vi "Update MLBox.vi"(8 "error in (no error)":errorcluster, 11 "Table View in":refnum<class "Table View.lvclass">) -> (0 "error out":errorcluster, 3 "Table View out":refnum<class "Table View.lvclass">)   [LabVIEW 2020, in "[V]Table View.lvlib" / "Table View.lvclass"]
uses:
  Table View.lvclass
  <vilib>/HUASUI/MulListBox/Type Definitions/Autosize Mode.ctl
  Table View.lvclass/Table View.ctl
  <vilib>/HUASUI/MulListBox/MListBox.lvclass/MListBox.ctl
  <vilib>/HUASUI/MulListBox/MListBox.lvclass
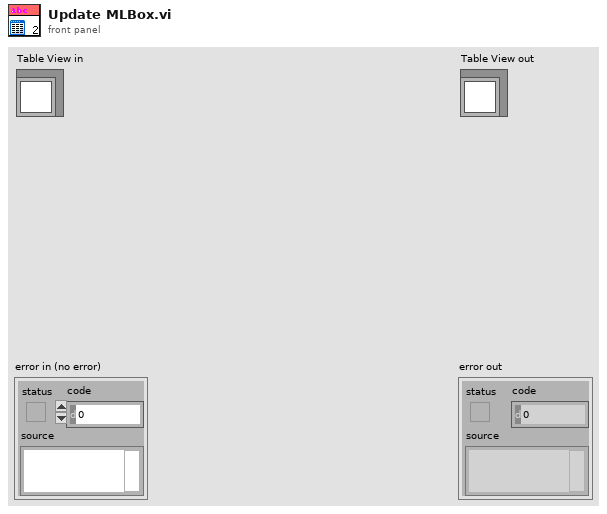
[diagram p1: front panel]
types:
  T1 = typedef "Autosize Mode.ctl" = enum16{"Header", "All Cells"}
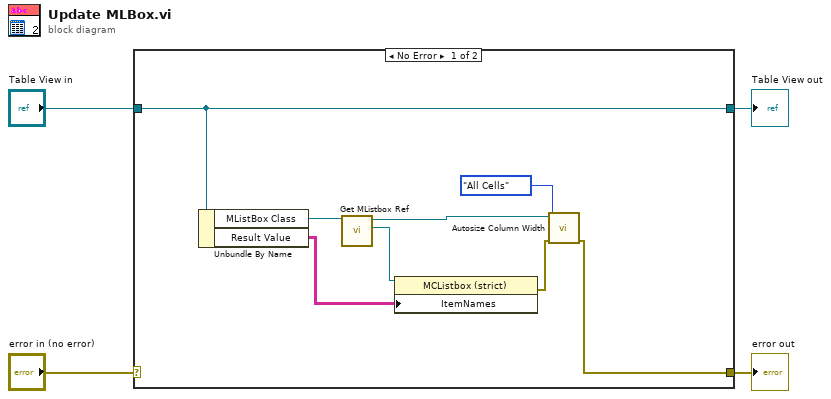
[diagram p0: block diagram]
diagram:
  n1 = case shown="No Error" "error in (no error)" {
    selector: "error in (no error)" -> [_ w14]
    tunnel: [w10 w14] -> w3
    tunnel: [w11 w13] -> w1
    tunnel: "Table View in" -> [w11 w13]
    frame No Error {
      n2 = Unbundle By Name(w11) -> ("MListBox Class"=w9:refnum<class "MListBox.lvclass">, "Result Value"=w8:string[][])
      n3 = call <vilib>:"Get MListbox Ref.vi"("Multicolumn ListBox in"=w9) -> ("MListbox Ref"=w7:refnum<vi>, "Multicolumn ListBox out"=w5:refnum<class "MListBox.lvclass">)  [unwired: 8 in, 1 out]
      n4 = property class="MCListbox (strict)"(reference=w7, "ItemNames"=w8) -> (error out=w6:errorcluster)  [unwired: 1 in, 1 out]
      n5 = call <vilib>:"Autosize Column Width.vi"("error in (no error)"=w6, "Autosize Mode"=Autosize_Mode."All Cells", "Multicolumn ListBox in"=w5) -> ("error out"=w10:errorcluster)  [unwired: 7 in, 1 out]
    }
    frame Error {
    }
  }
  "error out" <- w3
  "Table View out" <- w1
